vi "Cmd Get Integer Parameter Value (C).vi"(6 "error in (no error)":errorcluster, 7 "type":i32, 8 "parameter index":variant, 9 "command reference":T1) -> (0 "error out":errorcluster, 1 "value":i32, 3 "command reference out":T1)   [LabVIEW 2017, in "NI_Database_API.lvlib"]
doc: "Retrieves the value of the parameter specified by the <B>parameter index</B> input in the command or command-recordset. The <B>parameter index</B> can be either the zero-indexed position of the parameter in the command or the name of the parameter. Wire data to the <B>type</B> input to determine the polymorphic instance to use or manually select the instance."
uses:
  <vilib>/addons/database/NI_Database_API.lvlib
  <vilib>/addons/database/Command.llb/Cmd ObjectReference.ctl
  <vilib>/addons/database/_DB Variant To Data/Database Variant To Data.xnode
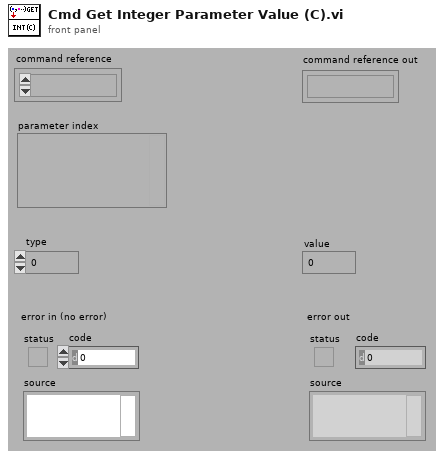
[diagram p1: front panel]
types:
  T1 = typedef "NI_Database_API.lvlib/Cmd ObjectReference.ctl" = refnum<k1>
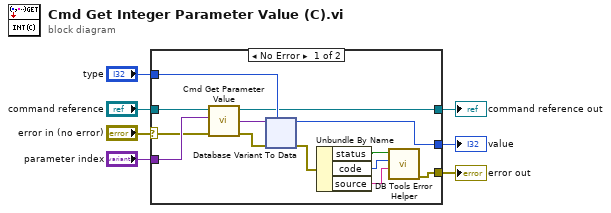
[diagram p0: block diagram]
diagram:
  n1 = case shown="No Error" "error in (no error)" {
    selector: "error in (no error)" -> [w8 w54]
    tunnel: "type" -> [w20 _]
    tunnel: [w19 _] -> w6
    tunnel: "command reference" -> [w18 w53]
    tunnel: "parameter index" -> [w17 _]
    tunnel: [w16 w53] -> w3
    tunnel: [w10 w54] -> w2
    frame No Error {
      n2 = call <vilib>:"Cmd Get Parameter Value.vi"("error in (no error)"=w8, "parameter index"=w17, "command reference"=w18) -> ("error out"=w14:errorcluster, "value"=w15:variant, "command reference out"=w16:T1)  [unwired: 2 out]
      n3 = xnode "Database Variant To Data"("database variant"=w15, "error in"=w14, "type"=w20) -> ("data"=w19:i32, "error out"=w11:errorcluster)
      n4 = Unbundle By Name(w11) -> ("status"=w13:bool, "code"=w12:i32, "source"=w9:string)
      n5 = call <vilib>:"DB Tools Error Helper.vi"("source"=w9, "code"=w12, "status"=w13) -> ("error out"=w10:errorcluster)  [unwired: 1 in, 7 out]
    }
    frame Error {
    }
  }
  "error out" <- w2
  "command reference out" <- w3
  "value" <- w6
